vi "testOpenCloseVeriStandConnection.vi"(8 "error in (no error)":errorcluster, 11 "TestCase in":refnum<class "VeriStandTestCaseSystemTests.lvclass">) -> (0 "error out":errorcluster, 3 "TestCase out":refnum<class "VeriStandTestCaseSystemTests.lvclass">)   [LabVIEW 2027, in "VeriStandTestCaseSystemTests.lvclass"]
uses:
  VeriStandTestCaseSystemTests.lvclass
  Source/VeriStandTestUtilities/SystemDefinitionInformation.ctl
  Source/VeriStandTestUtilities/TargetInformation.ctl
  Source/VeriStandTestUtilities/ChassisInformation.ctl
  <vilib>/NI VeriStand/Execution/Workspace/WorkspaceAPI.ctl
  C:/NetCoreDLL/NationalInstruments.VeriStand.ClientAPI.dll
  NetCoreDLL/NationalInstruments.VeriStand.ClientAPI.dll
  Source/VeriStandTestCase/VeriStandTestCase.lvclass
  C:/Program Files/National Instruments/LabVIEW 2027/vi.lib/addons/_JKI Toolkits/VI Tester/TestCase.llb/TestCase.lvclass
  <vilib>/addons/_JKI Toolkits/VI Tester/TestCase.llb/TestCase.lvclass
  Source/VeriStandTestUtilities/VeriStandTestUtilities.lvlib
  <vilib>/NI VeriStand/Execution/Workspace/NI_VS Workspace ExecutionAPI.lvlib
panel:
  out "WorkspaceManager":T1
  out "System Definition Information":T2
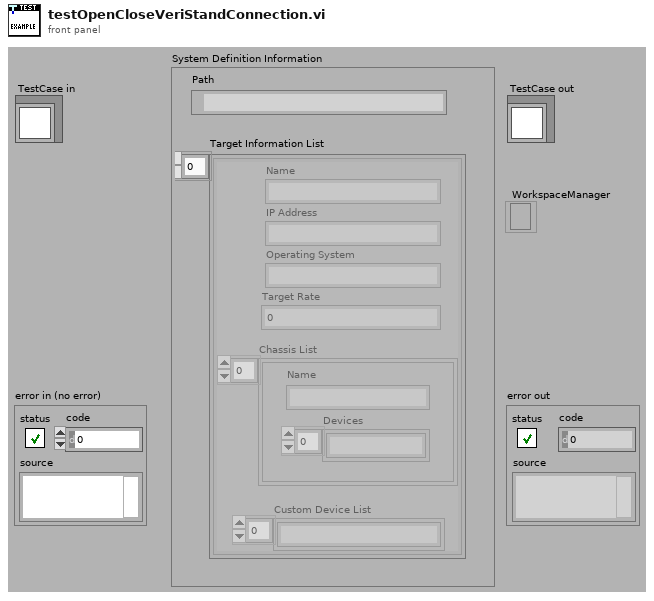
[diagram p1: front panel]
types:
  T1 = typedef "NI_VS Workspace ExecutionAPI.lvlib/WorkspaceAPI.ctl" = refnum<k39>
  T2 = typedef "VeriStandTestUtilities.lvlib/SystemDefinitionInformation.ctl" = cluster{"Path":path, "Target Information List":T3[]}
  T3 = typedef "VeriStandTestUtilities.lvlib/TargetInformation.ctl" = cluster{"Name":string, "IP Address":string, "Operating System":string, "Target Rate":dbl, "Chassis List":T4[], "Custom Device List":string[]}
  T4 = typedef "VeriStandTestUtilities.lvlib/ChassisInformation.ctl" = cluster{"Name":string, "Devices":string[]}
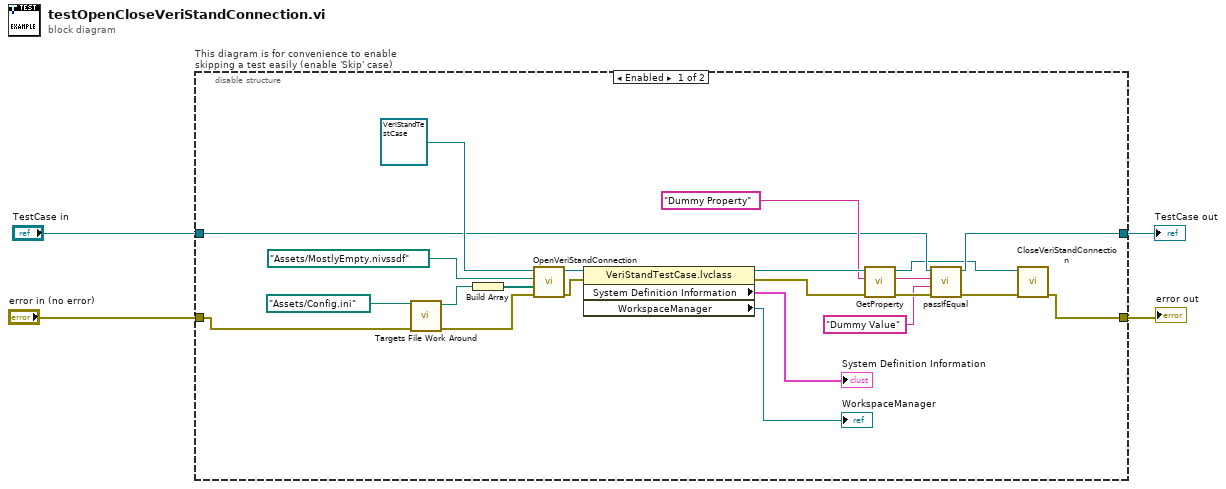
[diagram p0: block diagram]
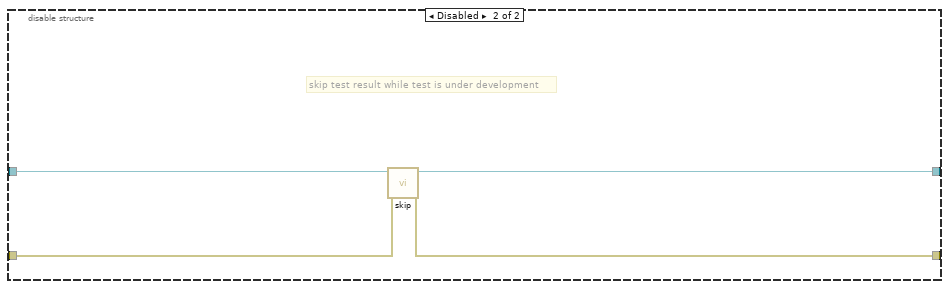
[diagram p2: hidden frame]
diagram:
  n1 = disable-structure "This diagram is for convenience to enable skipping a test easily (enable 'Skip' case)" shown="Enabled" {
    disable-tunnel: "TestCase in" -> [w14 w30]
    disable-tunnel: [w13 w28] -> w1
    disable-tunnel: [w25 w29] -> w3
    disable-tunnel: "error in (no error)" -> [w9 w27]
    frame Enabled {
      n2 = call "Targets File Work Around.vi"("error in (no error)"=w9, "overrides file in"=path "Assets/Config.ini" ("overrides files")) -> ("error out"=w8:errorcluster, "overrides file out"=w6:path)  [unwired: 8 in]
      n3 = Build Array(w6) -> (w7:path[])
      n4 = call-dynamic "OpenVeriStandConnection.vi"("error in (no error)"=w8, "overrides files"=w7, "System Definition File"=path "Assets/MostlyEmpty.nivssdf", "VeriStand Test Case in"=refnum<class "VeriStandTestCase.lvclass"> refnum) -> ("error out"=w22:errorcluster, "VeriStand Test Case out"=w23:refnum<class "VeriStandTestCase.lvclass">)  [unwired: 5 in, 1 out]
      n5 = property class="VeriStandTestCase.lvclass"(reference=w23, error in=w22) -> (reference out=w19:refnum<class "VeriStandTestCase.lvclass">, error out=w18:errorcluster, "System Definition Information"=→"System Definition Information":T2, "WorkspaceManager"=→"WorkspaceManager":T1)
      n6 = call "GetProperty.vi"("error in (no error)"=w18, "key"="Dummy Property", "VeriStandTestCase in"=w19) -> ("error out"=w16:errorcluster, "value"=w12:string, "VeriStandTestCase out"=w11:refnum<class "VeriStandTestCase.lvclass">)  [unwired: 6 in]
      n7 = call-dynamic "passIfEqual.vi"("error in (no error)"=w16, "y"="Dummy Value" ("key"), "x"=w12, "TestCase in"=w14) -> ("error out"=w15:errorcluster, "TestCase out"=w13:refnum<class "VeriStandTestCaseSystemTests.lvclass">)  [unwired: 6 in]
      n8 = call-dynamic "CloseVeriStandConnection.vi"("error in (no error)"=w15, "VeriStand Test Case in"=w11) -> ("error out"=w25:errorcluster)  [unwired: 8 in, 1 out]
    }
    frame Disabled {
      # "skip test result while test is under development"
      n9 = call <vilib>:"skip.vi"("error in (no error)"=w27, "TestCase in"=w30) -> ("error out"=w29:errorcluster, "TestCase out"=w28:refnum<class "VeriStandTestCaseSystemTests.lvclass">)  [unwired: 8 in]
    }
  }
  "error out" <- w3
  "TestCase out" <- w1
